vi "Brass.vi"(0 "Amount":fxp<+,8,0>, 4 "S/R":fxp<+,16,0>, 5 "1/Decay":fxp<+,16,0>, 6 "Sustain":fxp<+,16,0>, 7 "1/Attack":fxp<+,16,0>, 8 "Gate":bool, 9 "LFO":fxp<+/-,8,8>, 10 "M":fxp<+,32,32>, 11 "Trigger":bool) -> (3 "Brass Out":fxp<+/-,8,8>)   [LabVIEW 2015]
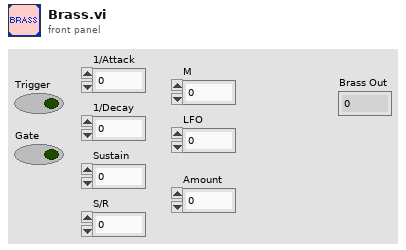
[diagram p1: front panel]
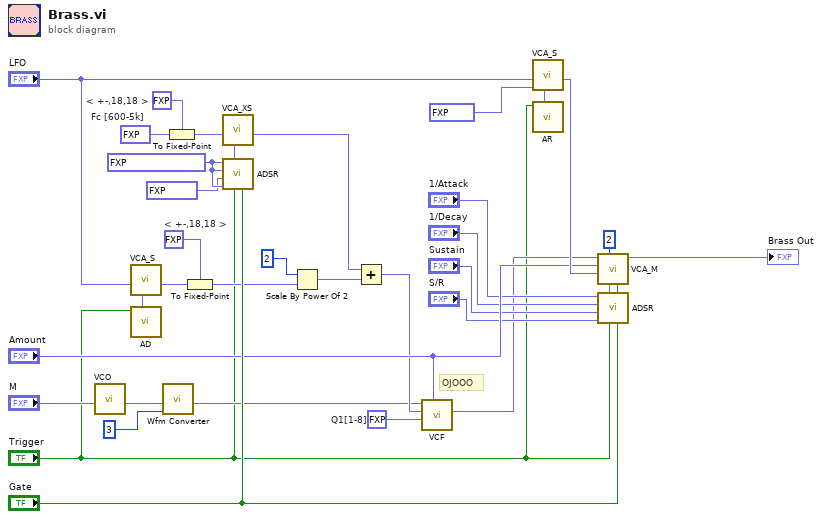
[diagram p0: block diagram]
diagram:
  w15 = fxp<+/-,32,16> 3000.0  # Fc [600-5k]
  w24 = fxp<+/-,18,18> 1.0  # Q1[1-8]
  w18 = fxp<+,16,0> 1.52587890625e-05 ("1/Attack")
  w16 = fxp<+/-,18,18> 0.0  # < +-,18,18 >
  w12 = fxp<+/-,18,18> 0.0  # < +-,18,18 >
  # "OJOOO"
  n1 = call "VCO.vi"("M"="M") -> ("Sine Sample"=w8:fxp<+/-,8,8>)  [unwired: 10 in]
  n2 = call "AD.vi"("Trigger"="Trigger") -> ("Sample Out"=w2:fxp<+,8,0>)  [unwired: 10 in]
  n3 = call "VCA_S.vi"("EG"=w2, "Sample In"="LFO") -> ("Sample Out"=w11:fxp<+/-,8,8>)  [unwired: 9 in]
  n4 = call "Wfm Converter.vi"("Select"=u8 3 ("select"), "Sample In"=w8) -> ("Sample Out"=w10:fxp<+/-,8,8>)  [unwired: 9 in]
  n5 = To Fixed-Point(fixed-point type=w16, number=w15) -> (fixed-point=w20:fxp<+/-,18,18>)
  n6 = To Fixed-Point(fixed-point type=w12, number=w11) -> (fixed-point=w13:fxp<+/-,18,18>)
  n7 = call "ADSR.vi"("Gate"="Gate", "Trigger"="Trigger", "S/R"=w18, "Sustain"=fxp<+,16,0> 0.8000030517578125 ("Sustain EG VCF"), "1/Decay"=w18, "1/Attack"=w18) -> ("Sample Out"=w19:fxp<+,8,0>)  [unwired: 4 in, 1 out]
  n8 = call "VCA_XS.vi"("EG"=w19, "Sample In"=w20) -> ("Sample Out"=w22:fxp<+/-,18,18>)  [unwired: 9 in]
  n9 = Scale By Power Of 2(n=u8 2 ("growl amount [0-2]"), x=w13) -> (x*2^n=w21:fxp<+/-,18,18>)
  n10 = Add(x=w22, y=w21) -> (x+y=w23:fxp<+/-,18,18>)
  n11 = call "VCF.vi"("Amount"="Amount", "Q1"=w24, "F1"=w23, "Sample In"=w10) -> ("LP Out"=w6:fxp<+/-,8,8>)  [unwired: 5 in, 2 out]
  n12 = call "AR.vi"("Trigger"="Trigger") -> ("Sample Out"=w1:fxp<+,8,0>)  [unwired: 10 in]
  n13 = call "VCA_S.vi"("EG"=w1, "Amount"=fxp<+,8,0> 0.28125 ("tremolo amount"), "Sample In"="LFO") -> ("Sample Out"=w33:fxp<+/-,8,8>)  [unwired: 8 in]
  n14 = call "ADSR.vi"("Gate"="Gate", "Trigger"="Trigger", "S/R"="S/R", "Sustain"="Sustain", "1/Decay"="1/Decay", "1/Attack"="1/Attack") -> ("Amount?"=w31:bool, "Sample Out"=w30:fxp<+,8,0>)  [unwired: 4 in]
  n15 = call "VCA_M.vi"("Amount?"=w31, "EG"=w30, "Scale"=i8 2, "LFO"=w33, "Amount"="Amount", "Sample In"=w6) -> ("Sample Out"=→"Brass Out":fxp<+/-,8,8>)  [unwired: 5 in]
